vi "Write Product Name.vi"(8 "error in (no error)":errorcluster, 10 "Product Name":string, 11 "Export in":refnum<class "Export.lvclass">) -> (0 "error out":errorcluster, 3 "Export out":refnum<class "Export.lvclass">)   [LabVIEW 2017, in "CL_G3_VIComponentBuilder.lvlib" / "Export.lvclass"]
uses:
  Export.lvclass
  Export.lvclass/Export.ctl
  Read Export Build Specification.vi
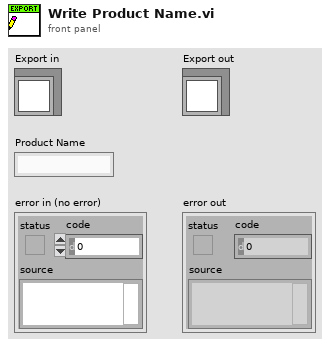
[diagram p1: front panel]
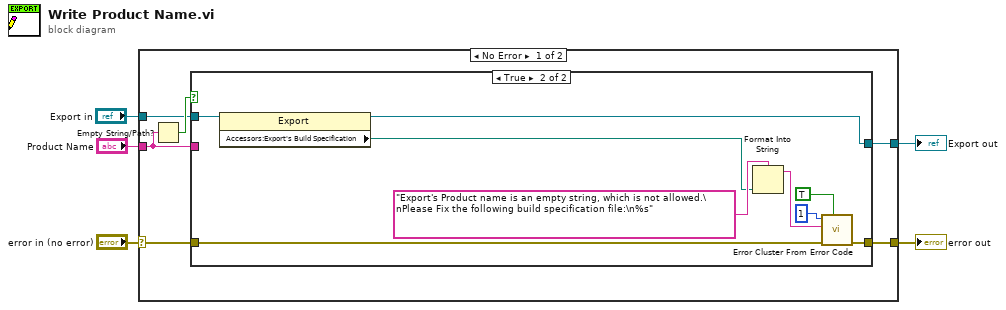
[diagram p0: block diagram]
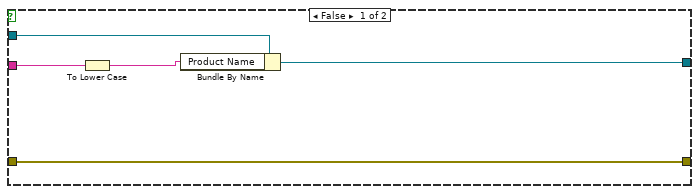
[diagram p2: hidden frame]
diagram:
  n1 = case shown="No Error" "error in (no error)" {
    selector: "error in (no error)" -> [w7 w26]
    tunnel: [w6 w26] -> w4
    tunnel: [w8 w27] -> w2
    tunnel: "Export in" -> [w9 w27]
    tunnel: "Product Name" -> [w10 _]
    frame No Error {
      n2 = Empty String/Path?(string/path=w10) -> (empty?=w11:bool)
      n3 = case shown="True" w11 {
        tunnel: w7 -> [w16 w24]
        tunnel: [w16 w17] -> w6
        tunnel: w9 -> [w15 w25]
        tunnel: [w14 w20] -> w8
        tunnel: w10 -> [w13 _]
        frame False {
          n4 = To Lower Case(string=w13) -> (all lower case string=w12:string)
          n5 = Bundle By Name(cluster=w15, "Product Name"=w12) -> (w14:refnum<class "Export.lvclass">)
        }
        frame True {
          n6 = property class="Export"(reference=w25) -> (reference out=w20:refnum<class "Export.lvclass">, "Accessors:Export's Build Specification"=w19:path)  [unwired: 1 in, 1 out]
          n7 = Format Into String(format string="Export's Product name is an empty string, which is not allowed.\nPlease Fix the following build specification file:\n%s" ("error message (\"\")"), w19) -> (resulting string=w18:string)  [unwired: 2 in, 1 out]
          n8 = call <vilib>:"Error Cluster From Error Code.vi"("show call chain? (False)"=TRUE, "error in (no error)"=w24, "error message (\"\")"=w18, "error code (0)"=1) -> ("error out"=w17:errorcluster)  [unwired: 5 in]
        }
      }
    }
    frame Error {
    }
  }
  "error out" <- w4
  "Export out" <- w2
